vi "Interface_Asset_Map Status.vi"(8 "error in (no error)":errorcluster, 11 "Grid in":refnum<class "Grid.lvclass">) -> (0 "error out":errorcluster, 3 "Grid out":refnum<class "Grid.lvclass">)   [LabVIEW 2015, in "Grid.lvclass"]
uses:
  Grid.lvclass
  Interface_Asset/Interface_Asset.lvclass
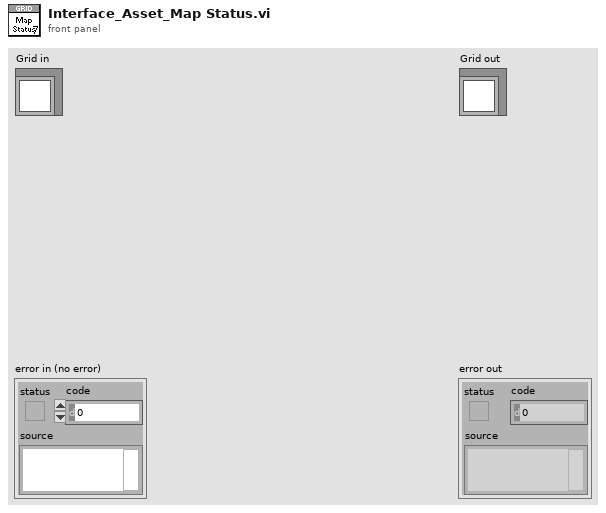
[diagram p1: front panel]
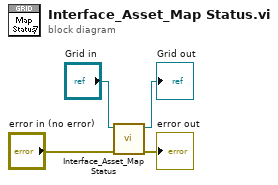
[diagram p0: block diagram]
diagram:
  n1 = call-parent "Interface_Asset_Map Status.vi"("error in (no error)"="error in (no error)", "Interface_Asset in"="Grid in") -> ("error out"=→"error out":errorcluster, "Interface_Asset out"=→"Grid out":refnum<class "Grid.lvclass">)  [unwired: 8 in]
